vi "report-test-started.vi"(8 "error in (no error)":errorcluster) -> (0 "error out":errorcluster)   [LabVIEW 2019]
uses:
  <vilib>/Rock Robotics/WPI/ThirdParty/JAS_Junk/TrajLib/Trajectory_Library.lvlib
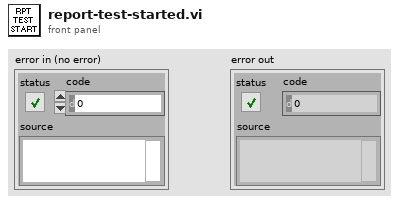
[diagram p1: front panel]
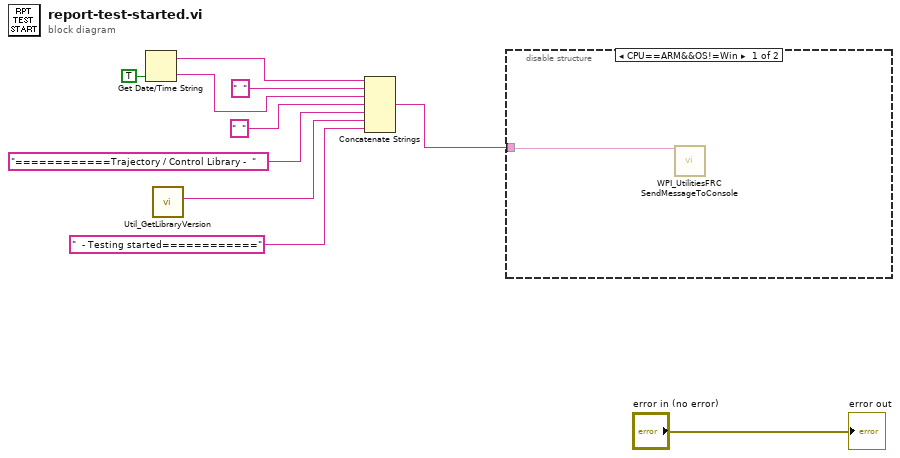
[diagram p0: block diagram]
diagram:
  n1 = Get Date/Time String(want seconds? (F)=TRUE) -> (date string=w8:string, time string=w6:string)  [unwired: 2 in]
  n2 = call <vilib>:"Util_GetLibraryVersion.vi"() -> ("TrajLibVersion"=w2:string)  [unwired: 11 in]
  n3 = Concatenate Strings(w8, "  " ("string"), w6, "  " ("string"), "============Trajectory / Control Library -  " ("string"), w2, "  - Testing started============" ("string")) -> (w3:string)
  n4 = disable-structure shown="CPU==ARM&&OS!=Win" {
    disable-tunnel: w3 -> [w11 _]
    frame condition #0 {
      n5 = call <vilib>:"WPI_UtilitiesFRC SendMessageToConsole.vi"("Message"=w11) -> ()  [unwired: 14 in, 1 out]
    }
    frame condition #1 (active) {
    }
  }
  "error out" <- "error in (no error)"
